vi "Waveform_Sync to End Time.vi"(6 "Open(t) Closed(f)":bool=TRUE, 8 "Error":errorcluster, 9 "tf":timestamp, 11 "Waveform":T1) -> (0 "Error Out":errorcluster, 2 "Final Time Out":timestamp, 3 "Waveform Out":T1)   [LabVIEW 2020]
uses:
  Universal Controls/Waveform_Data.ctl
  <vilib>/Waveform/WDTOps.llb/WDT Get Final Time Value DBL.vi
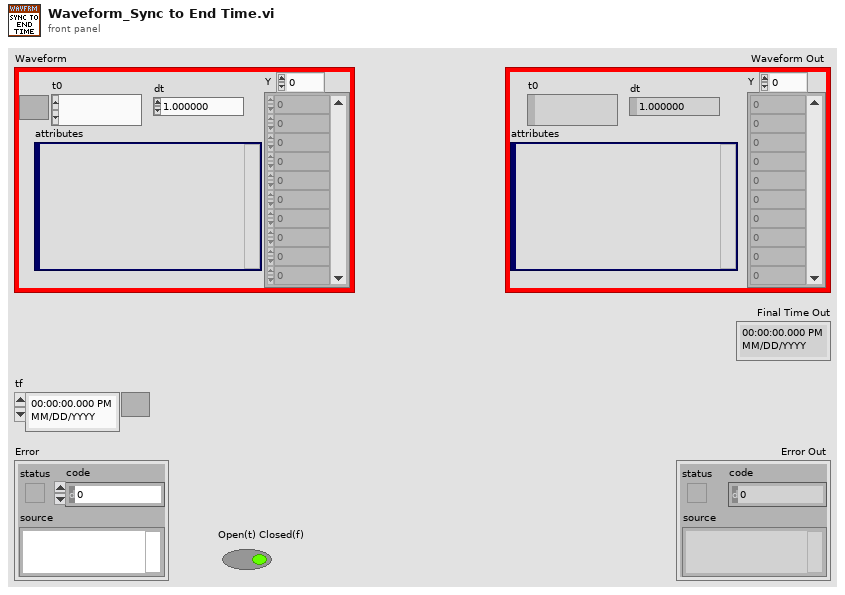
[diagram p1: front panel]
types:
  T1 = typedef "Waveform_Data.ctl" = waveform(dbl)
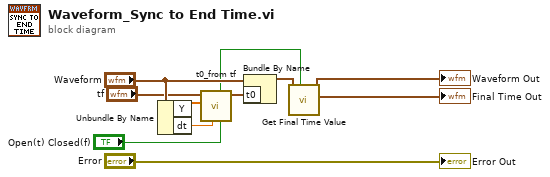
[diagram p0: block diagram]
diagram:
  n1 = Unbundle By Name("Waveform") -> ("Y"=w3:dbl[], "dt"=w2:dbl)
  n2 = call "t0_from tf.vi"("Open(t) Closed(f)"="Open(t) Closed(f)", "Dt"=w2, "Y"=w3, "Tf"="tf") -> ("New T0 Out"=w8:timestamp)  [unwired: 7 in]
  n3 = Bundle By Name(cluster="Waveform", "t0"=w8) -> (w7:T1)
  n4 = call-poly <vilib>:"Get Final Time Value.vi"("open interval? (T)"="Open(t) Closed(f)", "waveform in"=w7) -> ("tf"=→"Final Time Out":timestamp, "waveform out"=→"Waveform Out":waveform(dbl))  [unwired: 7 in, 1 out]
  "Error Out" <- "Error"
